vi "init runtime test.vi"() -> ()   [LabVIEW 2013, in "TEC tests.lvlib"]
uses:
  TEC tests.lvlib
  <vilib>/NI/Tag Bus Module Framework/channel/channel classification.ctl
  configuration/TEC configuration.lvclass
  execution/TEC runtime.lvclass
  configuration/TEC configuration.lvclass/TEC configuration.ctl
  <vilib>/NI/Tag Bus/tag/tag descriptor.lvclass/tag descriptor.ctl
  <vilib>/NI/Tag Bus Module Framework/channel/TBM channel.lvclass/TBM channel.ctl
  <vilib>/NI/Tag Bus/tag/read tag name.vi
  <vilib>/NI/Tag Bus/tag/read data type.vi
  <vilib>/NI/Tag Bus Module Framework/channel/Read channel classification.vi
  configuration/Write channels.vi
  <vilib>/NI/Tag Bus Module Framework/channel/TBM channel.lvclass
  <vilib>/NI/Tag Bus/dictionary/data dictionary.lvclass
  <vilib>/NI/Configuration Framework/serializable configuration/NISE_CEF_serializable configuration.lvclass
panel:
  out "tags found":bool
  out "no error":errorcluster
  out "expected execution settings":bool
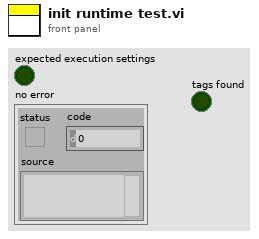
[diagram p1: front panel]
types:
  T1 = typedef "TBM channel.lvclass/channel classification.ctl" = enum16{"input data", "output data", "processing parameter", "processing result"}
  T2 = typedef "tag bus.lvlib/tag descriptor.lvclass/Data Type.ctl" = enum16{"Double", "Single", "I64", "I32", "I16", "I8", "U64", "U32", "U16", "U8", "Boolean", "String", "Array of Double", "Array of Single", "Array of I64", "Array of I32", "Array of I16", "Array of I8", "Array of U64", "Array of U32", "Array of U16", "Array of U8", "Array of Boolean", "Array of String"}
  T3 = typedef "TBM channel.lvclass/data tables.ctl" = cluster{"input data":T4, "processing parameter":T4, "processing result":T4, "output data":T4}
  T4 = typedef "tag bus.lvlib/dictionary table pair.ctl" = cluster{"data dictionary":refnum<class "data dictionary.lvclass">, "data table":T5}
  T5 = typedef "tag bus.lvlib/data table.lvlib/data table.ctl" = cluster{"Double":dbl[], "Single":sgl[], "I64":i64[], "I32":i32[], "I16":i16[], "I8":i8[], "U64":u64[], "U32":u32[], "U16":u16[], "U8":u8[], "Boolean":bool[], "String":string[], "Array of Double":cluster{"DBL Array":dbl[]}[], "Array of Single":cluster{"SGL Array":sgl[]}[], "Array of I64":cluster{"I64 Array":i64[]}[], "Array of I32":cluster{"I32 Array":i32[]}[], "Array of I16":cluster{"I16 Array":i16[]}[], "Array of I8":cluster{"I8 Array":i8[]}[], "Array of U64":cluster{"U64 Array":u64[]}[], "Array of U32":cluster{"U32 Array":u32[]}[], "Array of U16":cluster{"U16 Array":u16[]}[], "Array of U8":cluster{"U8 Array":u8[]}[], "Array of Boolean":cluster{"Boolean Array":bool[]}[], "Array of String":cluster{"String Array":string[]}[]}
  T6 = typedef "TBM module execution interface.lvclass/execution settings.ctl" = cluster{"reads inputs":bool, "processes data":bool, "writes outputs":bool}
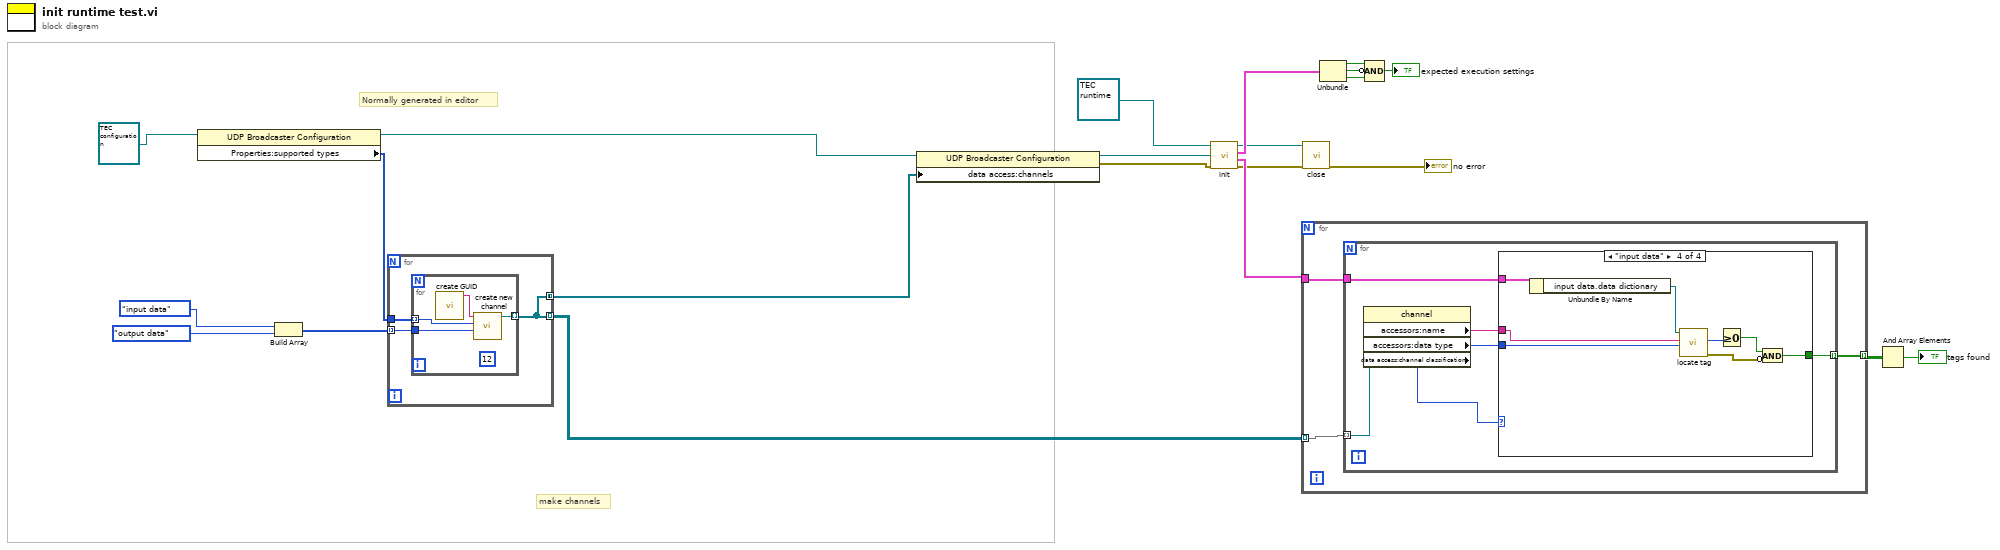
[diagram p0: block diagram]
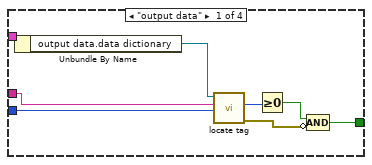
[diagram p2: hidden frame]
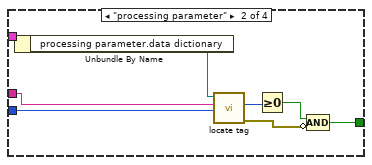
[diagram p3: hidden frame]
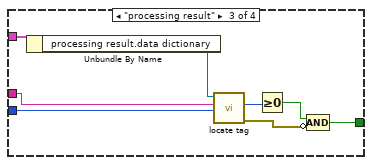
[diagram p4: hidden frame]
diagram:
  # "Normally generated in editor"
  # "make channels"
  n1 = property class="UDP Broadcaster Configuration"(reference=refnum<class "TEC configuration.lvclass"> refnum ("tag bus configurable plugin module configuration")) -> (reference out=w1:refnum<class "TEC configuration.lvclass">, "Properties:supported types"=w19:T2[])  [unwired: 1 in, 1 out]
  n2 = Build Array(channel_classification."input data" ("channel classification"), channel_classification."output data" ("channel classification")) -> (w20:T1[])
  n3 = for {
    tunnel: w20 -> [w25] mode=indexing
    tunnel: [w23] -> w12 mode=indexing
    tunnel: w19 -> [w24]
    tunnel: [w23] -> w2 mode=concatenating
    n4 = for {
      tunnel: w25 -> [w28]
      tunnel: [w29] -> w23 mode=indexing
      tunnel: w24 -> [w27] mode=indexing
      (unwired) 12
      n5 = call <vilib>:"create GUID.vi"() -> ("uuid"=w26:string)  [unwired: 11 in]
      n6 = call <vilib>:"create new channel.vi"("channel classification"=w28, "data type"=w27, "channel name"=w26) -> ("channel"=w29:refnum<class "TBM channel.lvclass">)  [unwired: 8 in]
    }
  }
  n7 = property class="UDP Broadcaster Configuration"(reference=w1, "data access:channels"=w2) -> (reference out=w3:refnum<class "TEC configuration.lvclass">, error out=w4:errorcluster)  [unwired: 1 in]
  n8 = call-dynamic "init.vi"("error in"=w4, "TBM module configuration in"=w3, "TEC runtime in"=refnum<class "TEC runtime.lvclass"> refnum ("tag bus configurable plugin module")) -> ("error out"=w9:errorcluster, "data allocations"=w18:T3, "execution settings"=w17:T6, "TEC runtime out"=w8:refnum<class "TEC runtime.lvclass">)  [unwired: 5 in]
  n9 = for {
    tunnel: w18 -> [w32]
    tunnel: w12 -> [w31] mode=indexing
    tunnel: [w30] -> w11 mode=indexing
    n10 = for {
      tunnel: w32 -> [w36]
      tunnel: w31 -> [w38] mode=indexing
      tunnel: [w33] -> w30 mode=indexing
      n11 = property class="channel"(reference=w38) -> ("accessors:name"=w34:string, "accessors:data type"=w35:T2, "data access:channel classification"=w37:T1)  [unwired: 1 in, 2 out]
      n12 = case shown="\"input data\"" w37 {
        tunnel: w36 -> [w46 w54 w62 w70]
        tunnel: w35 -> [w44 w52 w60 w68]
        tunnel: w34 -> [w43 w51 w59 w67]
        tunnel: [w39 w47 w55 w63] -> w33
        frame "output data" {
          n13 = Unbundle By Name(w46) -> ("output data.data dictionary"=w45:refnum<class "data dictionary.lvclass">)
          n14 = call <vilib>:"locate tag.vi"("data type"=w44, "name"=w43, "data dictionary in"=w45) -> ("error out"=w40:errorcluster, "index"=w42:i32)  [unwired: 6 in, 1 out]
          n15 = Greater Or Equal To 0?(x=w42) -> (x >= 0?=w41:bool)
          n16 = Compound Arithmetic op=AND(w41, invert w40) -> (w39:bool)
        }
        frame "processing parameter" {
          n17 = Unbundle By Name(w54) -> ("processing parameter.data dictionary"=w53:refnum<class "data dictionary.lvclass">)
          n18 = call <vilib>:"locate tag.vi"("data type"=w52, "name"=w51, "data dictionary in"=w53) -> ("error out"=w48:errorcluster, "index"=w50:i32)  [unwired: 6 in, 1 out]
          n19 = Greater Or Equal To 0?(x=w50) -> (x >= 0?=w49:bool)
          n20 = Compound Arithmetic op=AND(w49, invert w48) -> (w47:bool)
        }
        frame "processing result" {
          n21 = Unbundle By Name(w62) -> ("processing result.data dictionary"=w61:refnum<class "data dictionary.lvclass">)
          n22 = call <vilib>:"locate tag.vi"("data type"=w60, "name"=w59, "data dictionary in"=w61) -> ("error out"=w56:errorcluster, "index"=w58:i32)  [unwired: 6 in, 1 out]
          n23 = Greater Or Equal To 0?(x=w58) -> (x >= 0?=w57:bool)
          n24 = Compound Arithmetic op=AND(w57, invert w56) -> (w55:bool)
        }
        frame "input data" {
          n25 = Unbundle By Name(w70) -> ("input data.data dictionary"=w69:refnum<class "data dictionary.lvclass">)
          n26 = call <vilib>:"locate tag.vi"("data type"=w68, "name"=w67, "data dictionary in"=w69) -> ("error out"=w64:errorcluster, "index"=w66:i32)  [unwired: 6 in, 1 out]
          n27 = Greater Or Equal To 0?(x=w66) -> (x >= 0?=w65:bool)
          n28 = Compound Arithmetic op=AND(w65, invert w64) -> (w63:bool)
        }
      }
    }
  }
  n29 = call-dynamic "close.vi"("error in"=w9, "TEC runtime in"=w8) -> ("error out"=→"no error":errorcluster)  [unwired: 9 in]
  n30 = Unbundle(w17) -> ("reads inputs"=w16:bool, "processes data"=w14:bool, "writes outputs"=w15:bool)
  n31 = Compound Arithmetic op=AND(w16, invert w14, w15) -> (→"expected execution settings":bool)
  n32 = And Array Elements(Boolean array=w11) -> (logical AND=→"tags found":bool)
